vi "getFirstPixelPos(includingspace).vi"(6 "error in (no error)":errorcluster, 8 "y":dbl, 9 "delta":dbl=0.29999999999999716, 10 "min":dbl[](array[numeric]), 11 "max":dbl[](array[numeric])) -> (0 "delete":dbl[](array[numeric])=[0.0, -1800.0, 0.0], 1 "initialized array":dbl[](array[numeric]), 2 "totalLength":dbl, 3 "position":dbl[](array[numeric]), 4 "error out":errorcluster)   [LabVIEW 2020]
panel:
  out "position (colum)":dbl[](array[numeric])
  out "corrected width":dbl[](array[numeric])
  out "delta (colum)":dbl[](array[numeric])
  out "delta (energy)":dbl[](array[numeric])
  out "width (colum)":dbl[](array[numeric])
  out "1D-size":dbl[](array[numeric])
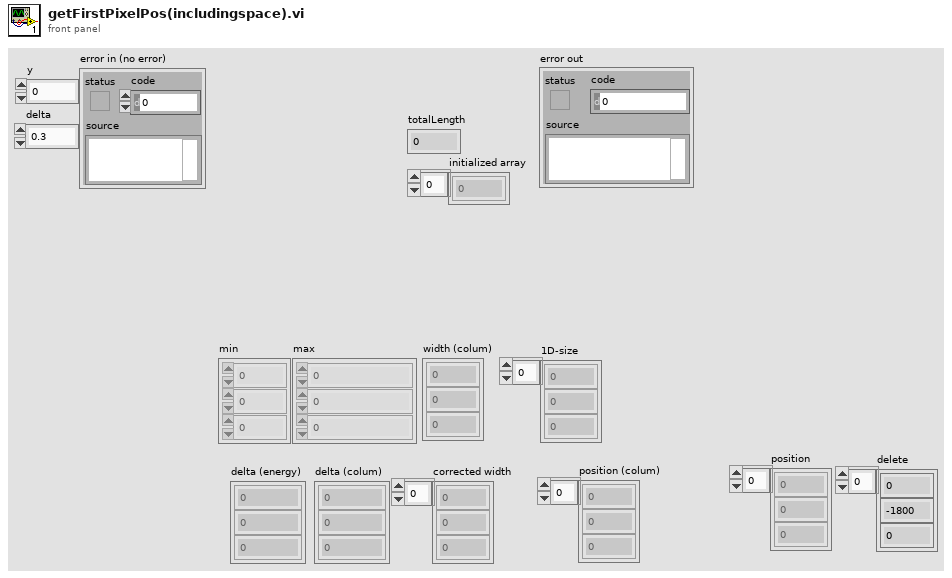
[diagram p1: front panel]
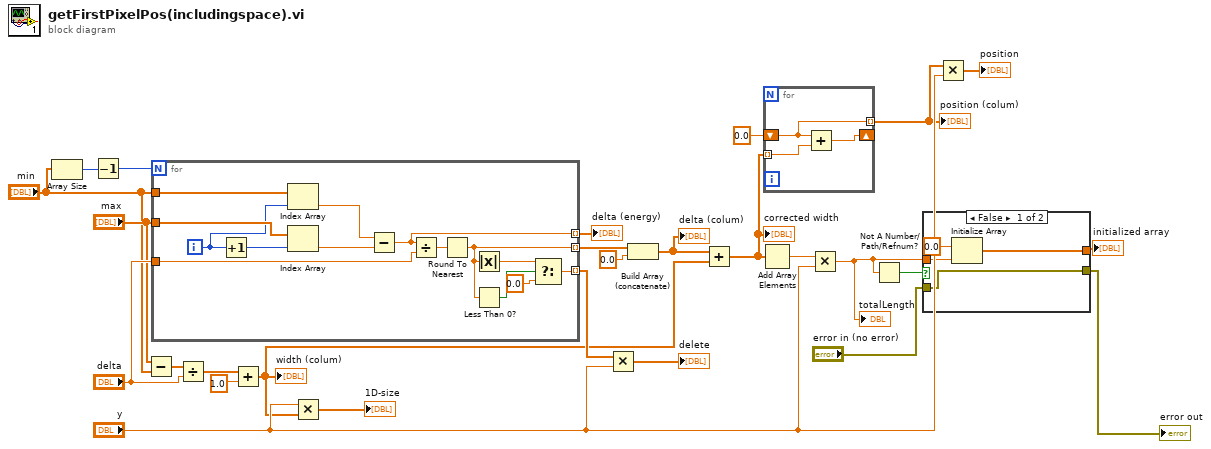
[diagram p0: block diagram]
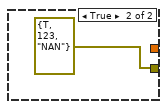
[diagram p2: hidden frame]
diagram:
  n1 = Array Size(array="min") -> (size(s)=w21:i32)
  n2 = Decrement(x=w21) -> (x-1=w20:i32)
  n3 = Subtract(x="max", y="min") -> (x-y=w27:dbl[])
  n4 = for {
    N: w20 -> [_]
    tunnel: "min" -> [w40]
    tunnel: "max" -> [w41]
    tunnel: "delta" -> [w35]
    tunnel: [w34] -> w26 mode=indexing
    tunnel: [w29] -> w19 mode=indexing
    tunnel: [w30] -> w15 mode=indexing
    i -> [w39]
    n5 = Increment(x=w39) -> (x+1=w38:i32)
    n6 = Index Array(array=w40, index=w39) -> (element=w37:dbl)
    n7 = Index Array(array=w41, index=w38) -> (element=w36:dbl)
    n8 = Subtract(x=w37, y=w36) -> (x-y=w34:dbl)
    n9 = Divide(x=w34, y=w35) -> (x/y=w33:dbl)
    n10 = Round To Nearest(number=w33) -> (nearest integer value=w29:dbl)
    n11 = Absolute Value(x=w29) -> (abs(x)=w28:dbl)
    n12 = Less Than 0?(x=w29) -> (x < 0?=w32:bool)
    n13 = Select(t=w28, s=w32, f=0.0) -> (s? t:f=w30:dbl)
  }
  "delta (energy)" <- w26
  n14 = Divide(x=w27, y="delta") -> (x/y=w7:dbl[])
  n15 = Add(x=w7, y=1.0) -> (x+y=w6:dbl[])
  "width (colum)" <- w6
  n16 = Multiply(x="y", y=w6) -> (x*y=→"1D-size":dbl[])
  n17 = Multiply(x=w15, y="y") -> (x*y=→"delete":dbl[])
  n18 = Build Array (concatenate)(w19, 0.0) -> (w16:dbl[])
  "delta (colum)" <- w16
  n19 = Add(x=w16, y=w6) -> (x+y=w13:dbl[])
  "corrected width" <- w13
  n20 = Add Array Elements(numeric array=w13) -> (sum=w12:dbl)
  n21 = for {
    tunnel: w13 -> [w44] mode=indexing
    shift-right: [w43] -> _
    shift-left: 0.0 -> [w42]
    tunnel: [w42] -> w9 mode=indexing
    n22 = Add(x=w42, y=w44) -> (x+y=w43:dbl)
  }
  "position (colum)" <- w9
  n23 = Multiply(x=w12, y="y") -> (x*y=w4:dbl)
  "totalLength" <- w4
  n24 = Not A Number/Path/Refnum?(number/path/refnum=w4) -> (NaN/Path/Refnum?=w3:bool)
  n25 = case shown="False" w3 {
    tunnel: w4 -> [w47 _]
    tunnel: [w46 _] -> w5
    tunnel: [w45 errorcluster {"status"=TRUE, "code"=123, "source"="NAN"} ("error out")] -> w2
    tunnel: "error in (no error)" -> [w45 _]
    frame False {
      n26 = Initialize Array(0.0, w47) -> (w46:dbl[])
    }
    frame True {
    }
  }
  "initialized array" <- w5
  "error out" <- w2
  n27 = Multiply(x=w9, y="y") -> (x*y=→"position":dbl[])
